vi "reverseArray.vi"(11 "angles: put 0 degree always as init angle":u16[](array[numeric])) -> (3 "Array out":u16[](array[numeric]))   [LabVIEW 2013]
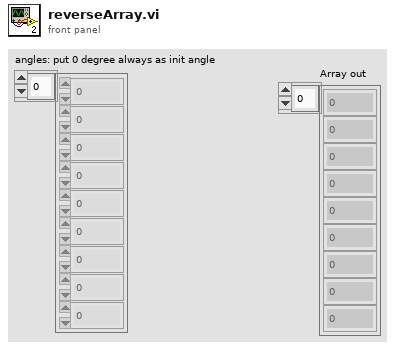
[diagram p1: front panel]
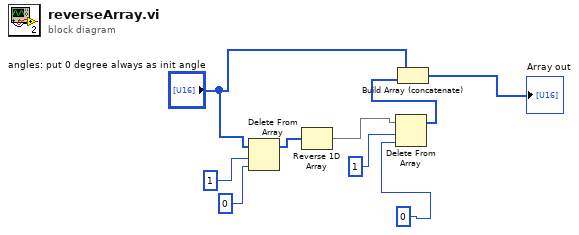
[diagram p0: block diagram]
diagram:
  n1 = Delete From Array(array="angles: put 0 degree always as init angle", length=1, index=0) -> (array with subset deleted=w1:u16[])  [unwired: 1 out]
  n2 = Reverse 1D Array(array=w1) -> (reversed array=w8:u16[])
  n3 = Delete From Array(array=w8, length=1, index=0) -> (array with subset deleted=w7:u16[])  [unwired: 1 out]
  n4 = Build Array (concatenate)("angles: put 0 degree always as init angle", w7) -> (→"Array out":u16[])
